vi "PH_SHS_Analysis_Calibrator.read calibration data.vi"(0 "file in":path, 1 "get latest from default directory":bool, 2 "get latest method depending":bool, 3 "Wanted Method":enum16{"automatic", "manual"}(ring), 4 "Certain Camera Instance?":string="N/A", 5 "error in (no error)":errorcluster) -> (14 "file out":path, 17 "SHS Analysis Calibration Data":T1, 19 "error out":errorcluster)   [LabVIEW 2014, in "PH_SHS_Analysis_Calibrator.lvlib"]
doc: "This VI reads out the calibration data file. If the input error is an error, the error is passing throung and nothing is done. If there is no incoming error, but an error ocours opening the file, reading the file or unpacking the data, error out is cleaned and the calibration data array is set to be empty. Otherwise the data are given out at Calibration data array."
uses:
  PH_SHS_Analysis_Calibrator.lvlib
  PH_SHS_Analysis_Calibrator.Analysis Calibration Data.ctl
  User/Eisenbarth/SHS_v4/SHS_Common/SHSReference.ctl
  User/Eisenbarth/SHS_v4/SHS_Common/ReferencePoint.ctl
  User/Eisenbarth/SHS_v4/SHS_Common/Rectangle.ctl
  User/Eisenbarth/SHS_v4/SHS_Common/Point.ctl
  PH_SHS_Analysis_Calibrator.Analysis Calibration Data - Version 1.ctl
  User/Eisenbarth/SHS_v4/SHS_Common/SHS_Common.lvlib
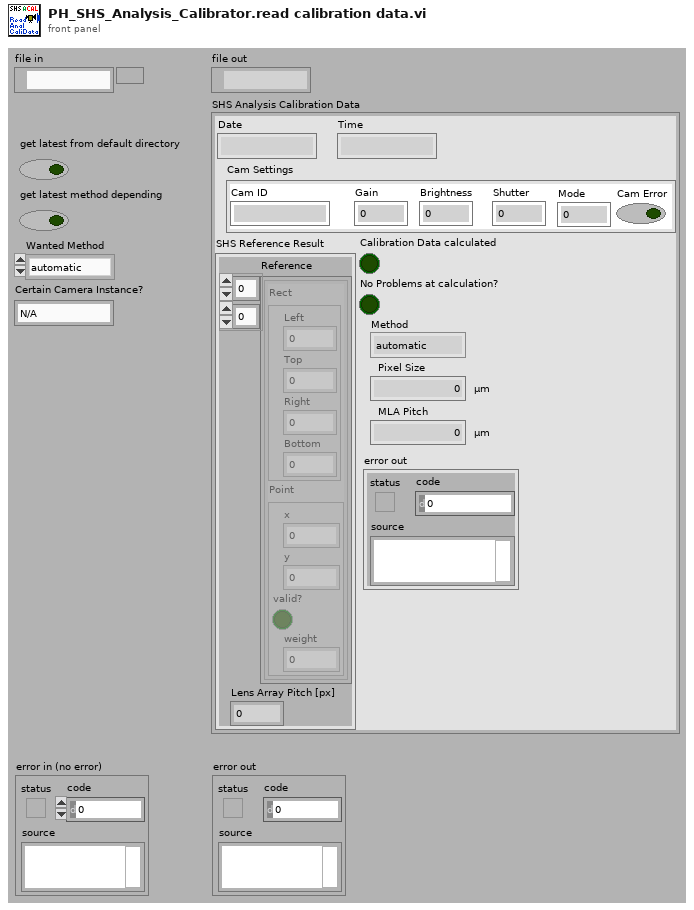
[diagram p1: front panel]
types:
  T1 = typedef "PH_SHS_Analysis_Calibrator.lvlib/PH_SHS_Analysis_Calibrator.Analysis Calibration Data.ctl" = cluster{"Date":string, "Time":string, "Cam Settings":cluster{"Cam ID":string, "Gain":dbl, "Brightness":dbl, "Shutter":dbl, "Cam Error":bool, "Mode":i32}, "SHS Reference Result":T2, "Pixel Size":dbl, "MLA Pitch":dbl, "Method":enum16{"automatic", "manual"}, "Calibration Data calculated":bool, "No Problems at calculation?":bool, "error out":errorcluster}
  T2 = typedef "SHS_Common.lvlib/SHSReference.ctl" = cluster{"Reference":T3[][], "Lens Array Pitch [px]":dbl}
  T3 = typedef "SHS_Common.lvlib/ReferencePoint.ctl" = cluster{"Rect":T4, "Point":T5}
  T4 = typedef "SHS_Common.lvlib/Rectangle.ctl" = cluster{"Left":i32, "Top":i32, "Right":i32, "Bottom":i32}
  T5 = typedef "SHS_Common.lvlib/Point.ctl" = cluster{"x":dbl, "y":dbl, "valid?":bool, "weight":dbl}
  T6 = typedef "PH_SHS_Analysis_Calibrator.lvlib/PH_SHS_Analysis_Calibrator.Analysis Calibration Data - Version 1.ctl" = cluster{"Date":string, "Time":string, "Cam Settings":cluster{"Serial Number":dbl, "Gain":i32, "Brightness":i32, "Shutter":i32, "Cam Error":bool, "Mode":i32}, "SHS Reference Result":T2, "Pixel Size [µm]":dbl, "MLA Pitch [µm]":dbl, "Method":enum16{"automatic", "manual"}, "Calibration Data calculated":bool, "No Problems at calculation?":bool, "error out":errorcluster}
  T7 = enum16{"open", "replace", "create", "open or create", "replace or create", "replace or create with confirmation"}
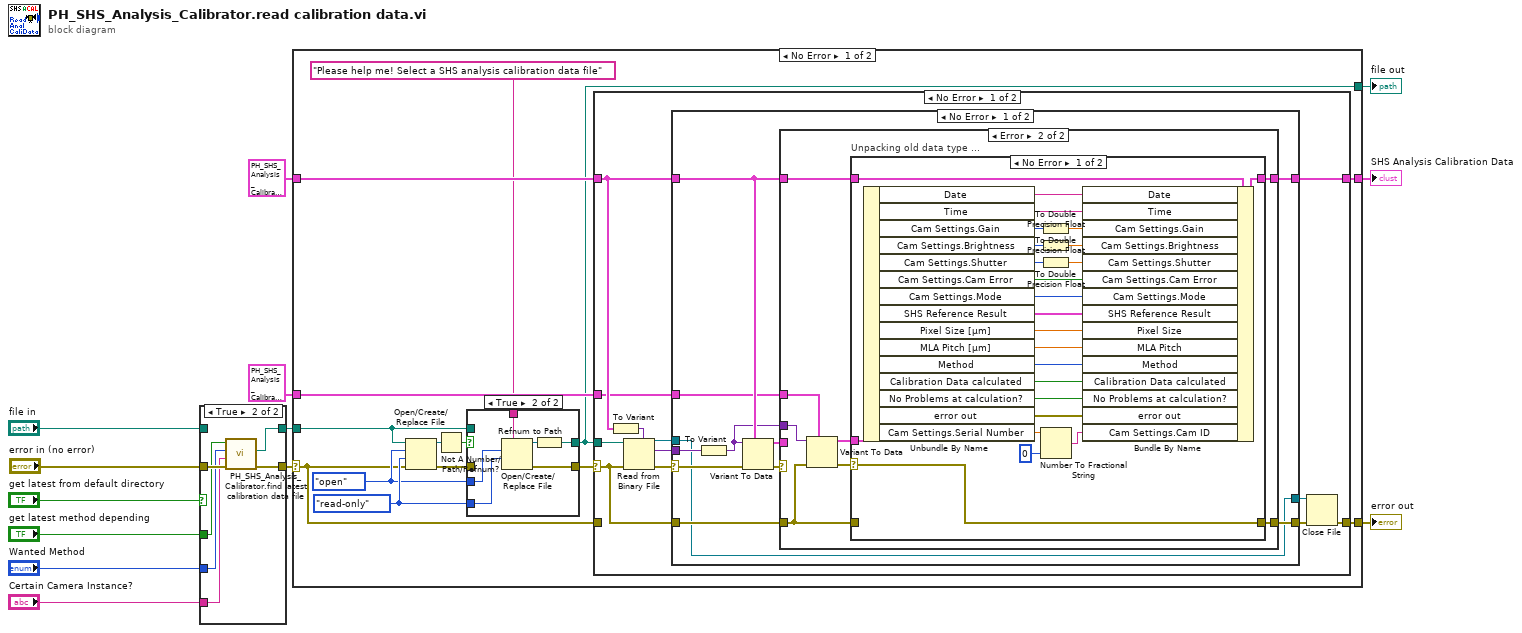
[diagram p0: block diagram]
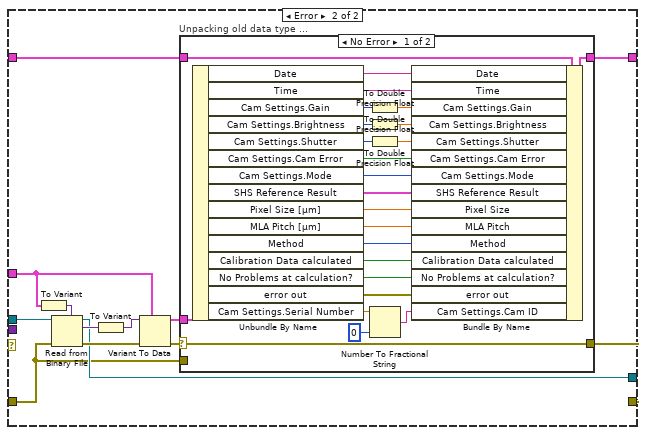
[diagram p5: hidden frame]
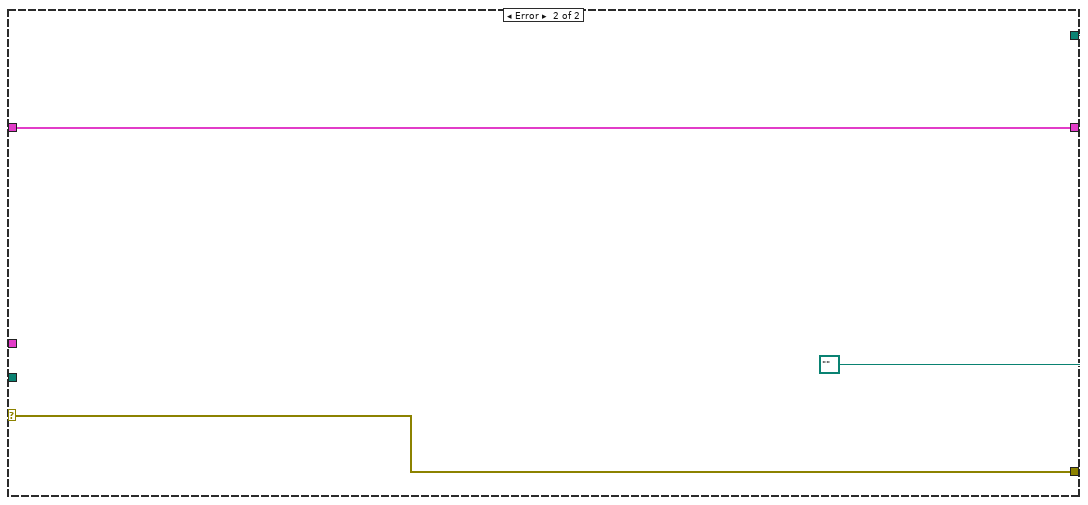
[diagram p9: hidden frame]
diagram:
  n1 = case shown="True" "get latest from default directory" {
    tunnel: "error in (no error)" -> [w14 w21]
    tunnel: [w14 w20] -> w11
    tunnel: "get latest method depending" -> [_ w18]
    tunnel: "Wanted Method" -> [_ w17]
    tunnel: "Certain Camera Instance?" -> [_ w16]
    tunnel: "file in" -> [w15 _]
    tunnel: [w15 w19] -> w5
    frame False {
    }
    frame True {
      n2 = call "PH_SHS_Analysis_Calibrator.find latest calibration data file.vi"("error in (no error)"=w21, "Certain Camera Instance?"=w16, "Wanted Method"=w17, "get latest method depending"=w18) -> ("error out"=w20:errorcluster, "latest file"=w19:path)  [unwired: 1 in, 1 out]
    }
  }
  n3 = case shown="No Error" w11 {
    selector: w11 -> [w26 w146]
    tunnel: [w28 w146] -> w13
    tunnel: [w27 w145] -> w1
    tunnel: T1 {"Date"="", "Time"="", "Cam Settings"={"Cam ID"="", "Gain"=0.0, "Brightness"=0.0, "Shutter"=0.0, "Cam Error"=FALSE, "Mode"=0}, "SHS Reference Result"={"Reference"=[], "Lens Array Pitch [px]"=0.0}, "Pixel Size"=0.0, "MLA Pitch"=0.0, "Method"=enum."automatic", "Calibration Data calculated"=FALSE, "No Problems at calculation?"=FALSE, "error out"={"status"=FALSE, "code"=0, "source"=""}} ("SHS Analysis Calibration Data") -> [w25 w145]
    tunnel: w5 -> [w32 _]
    tunnel: [w23 path "" ("latest file")] -> w4
    tunnel: T6 {"Date"="", "Time"="", "Cam Settings"={"Serial Number"=0.0, "Gain"=0, "Brightness"=0, "Shutter"=0, "Cam Error"=FALSE, "Mode"=0}, "SHS Reference Result"={"Reference"=[], "Lens Array Pitch [px]"=0.0}, "Pixel Size [µm]"=0.0, "MLA Pitch [µm]"=0.0, "Method"=enum."automatic", "Calibration Data calculated"=FALSE, "No Problems at calculation?"=FALSE, "error out"={"status"=FALSE, "code"=0, "source"=""}} ("SHS Analysis Calibration Data - Version 1") -> [w24 _]
    frame No Error {
      w31 = enum16{"read/write", "read-only", "write-only"}."read-only" ("access (0:read/write)")
      w30 = T7."open" ("operation (0:open)")
      n4 = Open/Create/Replace File(file path (use dialog)=w32, error in=w26, operation (0:open)=w30, access (0:read/write)=w31) -> (refnum out=w35:refnum<file>, error out=w34:errorcluster)  [unwired: 2 in, 1 out]
      n5 = Not A Number/Path/Refnum?(number/path/refnum=w35) -> (NaN/Path/Refnum?=w33:bool)
      n6 = case shown="True" w33 {
        tunnel: w34 -> [w137 _]
        tunnel: [w137 w143] -> w29
        tunnel: [w136 w139] -> w23
        tunnel: w32 -> [w136 _]
        tunnel: w31 -> [_ w141]
        tunnel: w30 -> [_ w140]
        tunnel: "Please help me! Select a SHS analysis calibration data file" ("prompt (Open existing file)") -> [_ w138]
        frame False {
        }
        frame True {
          n7 = Open/Create/Replace File(prompt=w138, operation (0:open)=w140, access (0:read/write)=w141) -> (refnum out=w142:refnum<file>, error out=w143:errorcluster)  [unwired: 3 in, 1 out]
          n8 = Refnum to Path(1:w142) -> (0:w139:path)
        }
      }
      n9 = case shown="No Error" w29 {
        selector: w29 -> [w40 _]
        tunnel: w23 -> [w47 _]
        tunnel: [w39 w135] -> w28
        tunnel: [w43 w134] -> w27
        tunnel: w25 -> [w44 w134]
        tunnel: w26 -> [_ w135]
        tunnel: w24 -> [w41 _]
        frame No Error {
          n10 = To Variant(anything=w44) -> (Variant=w45:variant)
          n11 = Read from Binary File(5:w45, 8:w40, 11:w47) -> (0:w42:errorcluster, 2:w46:variant, 3:w37:refnum<file>)  [unwired: 3 in, 1 out]
          n12 = case shown="No Error" w42 {
            selector: w42 -> [w52 _]
            tunnel: w46 -> [w58 _]
            tunnel: w44 -> [w56 w96]
            tunnel: [w55 w97] -> w43
            tunnel: [w53 w99] -> w38
            tunnel: w40 -> [w51 w98]
            tunnel: w41 -> [w48 w103]
            tunnel: w37 -> [w50 w102]
            tunnel: [w50 w101] -> w36
            frame No Error {
              n13 = To Variant(anything=w58) -> (Variant=w49:variant)
              n14 = Variant To Data(error in=w52, type=w56, Variant=w49) -> (data=w54:T1, error out=w57:errorcluster)
              n15 = case shown="Error" w57 {
                selector: w57 -> [w59 _]
                tunnel: w56 -> [_ w62]
                tunnel: [w60 w61] -> w55
                tunnel: w54 -> [w60 _]
                tunnel: [w59 w64] -> w53
                tunnel: w51 -> [_ w65]
                tunnel: w49 -> [_ w68]
                tunnel: w48 -> [_ w67]
                frame No Error {
                }
                frame Error {
                  n16 = Variant To Data(error in=w65, type=w67, Variant=w68) -> (data=w63:T6, error out=w66:errorcluster)
                  n17 = case "Unpacking old data type ..." shown="No Error" w66 {
                    selector: w66 -> [w92 _]
                    tunnel: [w92 w94] -> w64
                    tunnel: w65 -> [_ w94]
                    tunnel: [w90 w93] -> w61
                    tunnel: w62 -> [w91 w93]
                    tunnel: w63 -> [w89 _]
                    frame No Error {
                      n18 = Unbundle By Name(w89) -> ("Date"=w88:string, "Time"=w83:string, "Cam Settings.Gain"=w79:i32, "Cam Settings.Brightness"=w80:i32, "Cam Settings.Shutter"=w81:i32, "Cam Settings.Cam Error"=w82:bool, "Cam Settings.Mode"=w84:i32, "SHS Reference Result"=w85:T2, "Pixel Size [µm]"=w86:dbl, "MLA Pitch [µm]"=w87:dbl, "Method"=w73:enum16{"automatic", "manual"}, "Calibration Data calculated"=w72:bool, "No Problems at calculation?"=w71:bool, "error out"=w70:errorcluster, "Cam Settings.Serial Number"=w75:dbl)
                      n19 = To Double Precision Float(number=w79) -> (double precision float=w78:dbl)
                      n20 = To Double Precision Float(number=w80) -> (double precision float=w77:dbl)
                      n21 = To Double Precision Float(number=w81) -> (double precision float=w76:dbl)
                      n22 = Number To Fractional String(number=w75, precision (6)=i16 0) -> (F-format string=w74:string)  [unwired: 2 in]
                      n23 = Bundle By Name(cluster=w91, "Date"=w88, "Time"=w83, "Cam Settings.Gain"=w78, "Cam Settings.Brightness"=w77, "Cam Settings.Shutter"=w76, "Cam Settings.Cam Error"=w82, "Cam Settings.Mode"=w84, "SHS Reference Result"=w85, "Pixel Size"=w86, "MLA Pitch"=w87, "Method"=w73, "Calibration Data calculated"=w72, "No Problems at calculation?"=w71, "error out"=w70, "Cam Settings.Cam ID"=w74) -> (w90:T1)
                    }
                    frame Error {
                    }
                  }
                }
              }
            }
            frame Error {
              n24 = To Variant(anything=w103) -> (Variant=w106:variant)
              n25 = Read from Binary File(5:w106, 8:w98, 11:w102) -> (0:w107:errorcluster, 2:w104:variant, 3:w101:refnum<file>)  [unwired: 3 in, 1 out]
              n26 = To Variant(anything=w104) -> (Variant=w105:variant)
              n27 = Variant To Data(error in=w107, type=w103, Variant=w105) -> (data=w95:T6, error out=w100:errorcluster)
              n28 = case "Unpacking old data type ..." shown="No Error" w100 {
                selector: w100 -> [w131 _]
                tunnel: [w131 w133] -> w99
                tunnel: w98 -> [_ w133]
                tunnel: [w129 w132] -> w97
                tunnel: w96 -> [w130 w132]
                tunnel: w95 -> [w128 _]
                frame No Error {
                  n29 = Unbundle By Name(w128) -> ("Date"=w127:string, "Time"=w122:string, "Cam Settings.Gain"=w118:i32, "Cam Settings.Brightness"=w119:i32, "Cam Settings.Shutter"=w120:i32, "Cam Settings.Cam Error"=w121:bool, "Cam Settings.Mode"=w123:i32, "SHS Reference Result"=w124:T2, "Pixel Size [µm]"=w125:dbl, "MLA Pitch [µm]"=w126:dbl, "Method"=w112:enum16{"automatic", "manual"}, "Calibration Data calculated"=w111:bool, "No Problems at calculation?"=w110:bool, "error out"=w109:errorcluster, "Cam Settings.Serial Number"=w114:dbl)
                  n30 = To Double Precision Float(number=w118) -> (double precision float=w117:dbl)
                  n31 = To Double Precision Float(number=w119) -> (double precision float=w116:dbl)
                  n32 = To Double Precision Float(number=w120) -> (double precision float=w115:dbl)
                  n33 = Number To Fractional String(number=w114, precision (6)=i16 0) -> (F-format string=w113:string)  [unwired: 2 in]
                  n34 = Bundle By Name(cluster=w130, "Date"=w127, "Time"=w122, "Cam Settings.Gain"=w117, "Cam Settings.Brightness"=w116, "Cam Settings.Shutter"=w115, "Cam Settings.Cam Error"=w121, "Cam Settings.Mode"=w123, "SHS Reference Result"=w124, "Pixel Size"=w125, "MLA Pitch"=w126, "Method"=w112, "Calibration Data calculated"=w111, "No Problems at calculation?"=w110, "error out"=w109, "Cam Settings.Cam ID"=w113) -> (w129:T1)
                }
                frame Error {
                }
              }
            }
          }
          n35 = Close File(refnum=w36, error in=w38) -> (error out=w39:errorcluster)  [unwired: 1 out]
        }
        frame Error {
        }
      }
    }
    frame Error {
    }
  }
  "error out" <- w13
  "SHS Analysis Calibration Data" <- w1
  "file out" <- w4
